vi "AverageLiveSpectra.vi"(6 "Magnitude Averages":u8(slide) scale=1.0..10.0, 9 "old reading":waveform(dbl)[](graph), 10 "new reading":waveform(dbl)[](graph), 11 "Settings":T1 {"Ch_2" min=1 step=1; "Ch_1" min=1 max=100 step=1; "Trigger" items=["Hammer (force)", "Self-tap", "Spacebar"]; "Bandwidth" items=["1 kHz"=1, "5 kHz"=5, "10 kHz"=10, "25 kHz"=25, "50 kHz"=50, "100 kHz"=100]; "High Pass" items=["Off", "13 Hz", "104 Hz"]; "Range" items=["10 mm/s"=1, "20 mm/s"=2, "50 mm/s"=5, "100 mm/s"=10, "200 mm/s"=20, "500 mm/s"=50, "1 m/s"=100, "2 m/s"=200]; "Output" items=["Accelerometer", "Speed (from acceleration)", "Microphone", "Vibrometer", "Piezo"]; "Voltage Cal" format="%#_13g"; "Ch2 Gain" format="%#_13g"; "Ch1 Gain" format="%#_13g"; "Double bounce" min=0.0; "Mic cutoff" min=0.0 format="%#_4g"; "Hammer cutoff" min=0.0 format="%#_4g"; "Freq resolution" min=0.0; "Pre-trigger (s)" format="%#_13g"; "Date" format="%<%H:%M\n%d/%m/%y>T"; "resolution" items=["16 bit"=16, "24 bit"=24, "32 bit"=32]; "Sampling rate" items=["22050 samp/s"=22050, "44100 samp/s"=44100, "48000 samp/s"=48000]}) -> (0 "Hammer":waveform(dbl)(graph), 1 "FIFO out":waveform(dbl)[](array[waveform]), 2 "average spectrum":waveform(dbl), 3 "Power Spectrum":waveform(dbl)(graph), 4 "Microphone":waveform(dbl)(graph), 5 "Cal Hammer":waveform(dbl)[](graph), 7 "cal Mic":waveform(dbl)[](graph))   [LabVIEW 2022 SP3]
uses:
  PreferencesControl.ctl
  <vilib>/Analysis/NI_AALPro.lvlib
panel:
  out "Ch 1":waveform(dbl)(graph)
  # "Hz"
  # "dB"
  # "dB"
  # "sec"
  # "sec"
  # "mV/Pa"
  # "mV/m/s2"
  # "mV/mm/s"
  # "V/N"
  # "sec"
  # "sec"
  # "mV/N"
  # "a.u."
  # "a.u."
  # "sec"
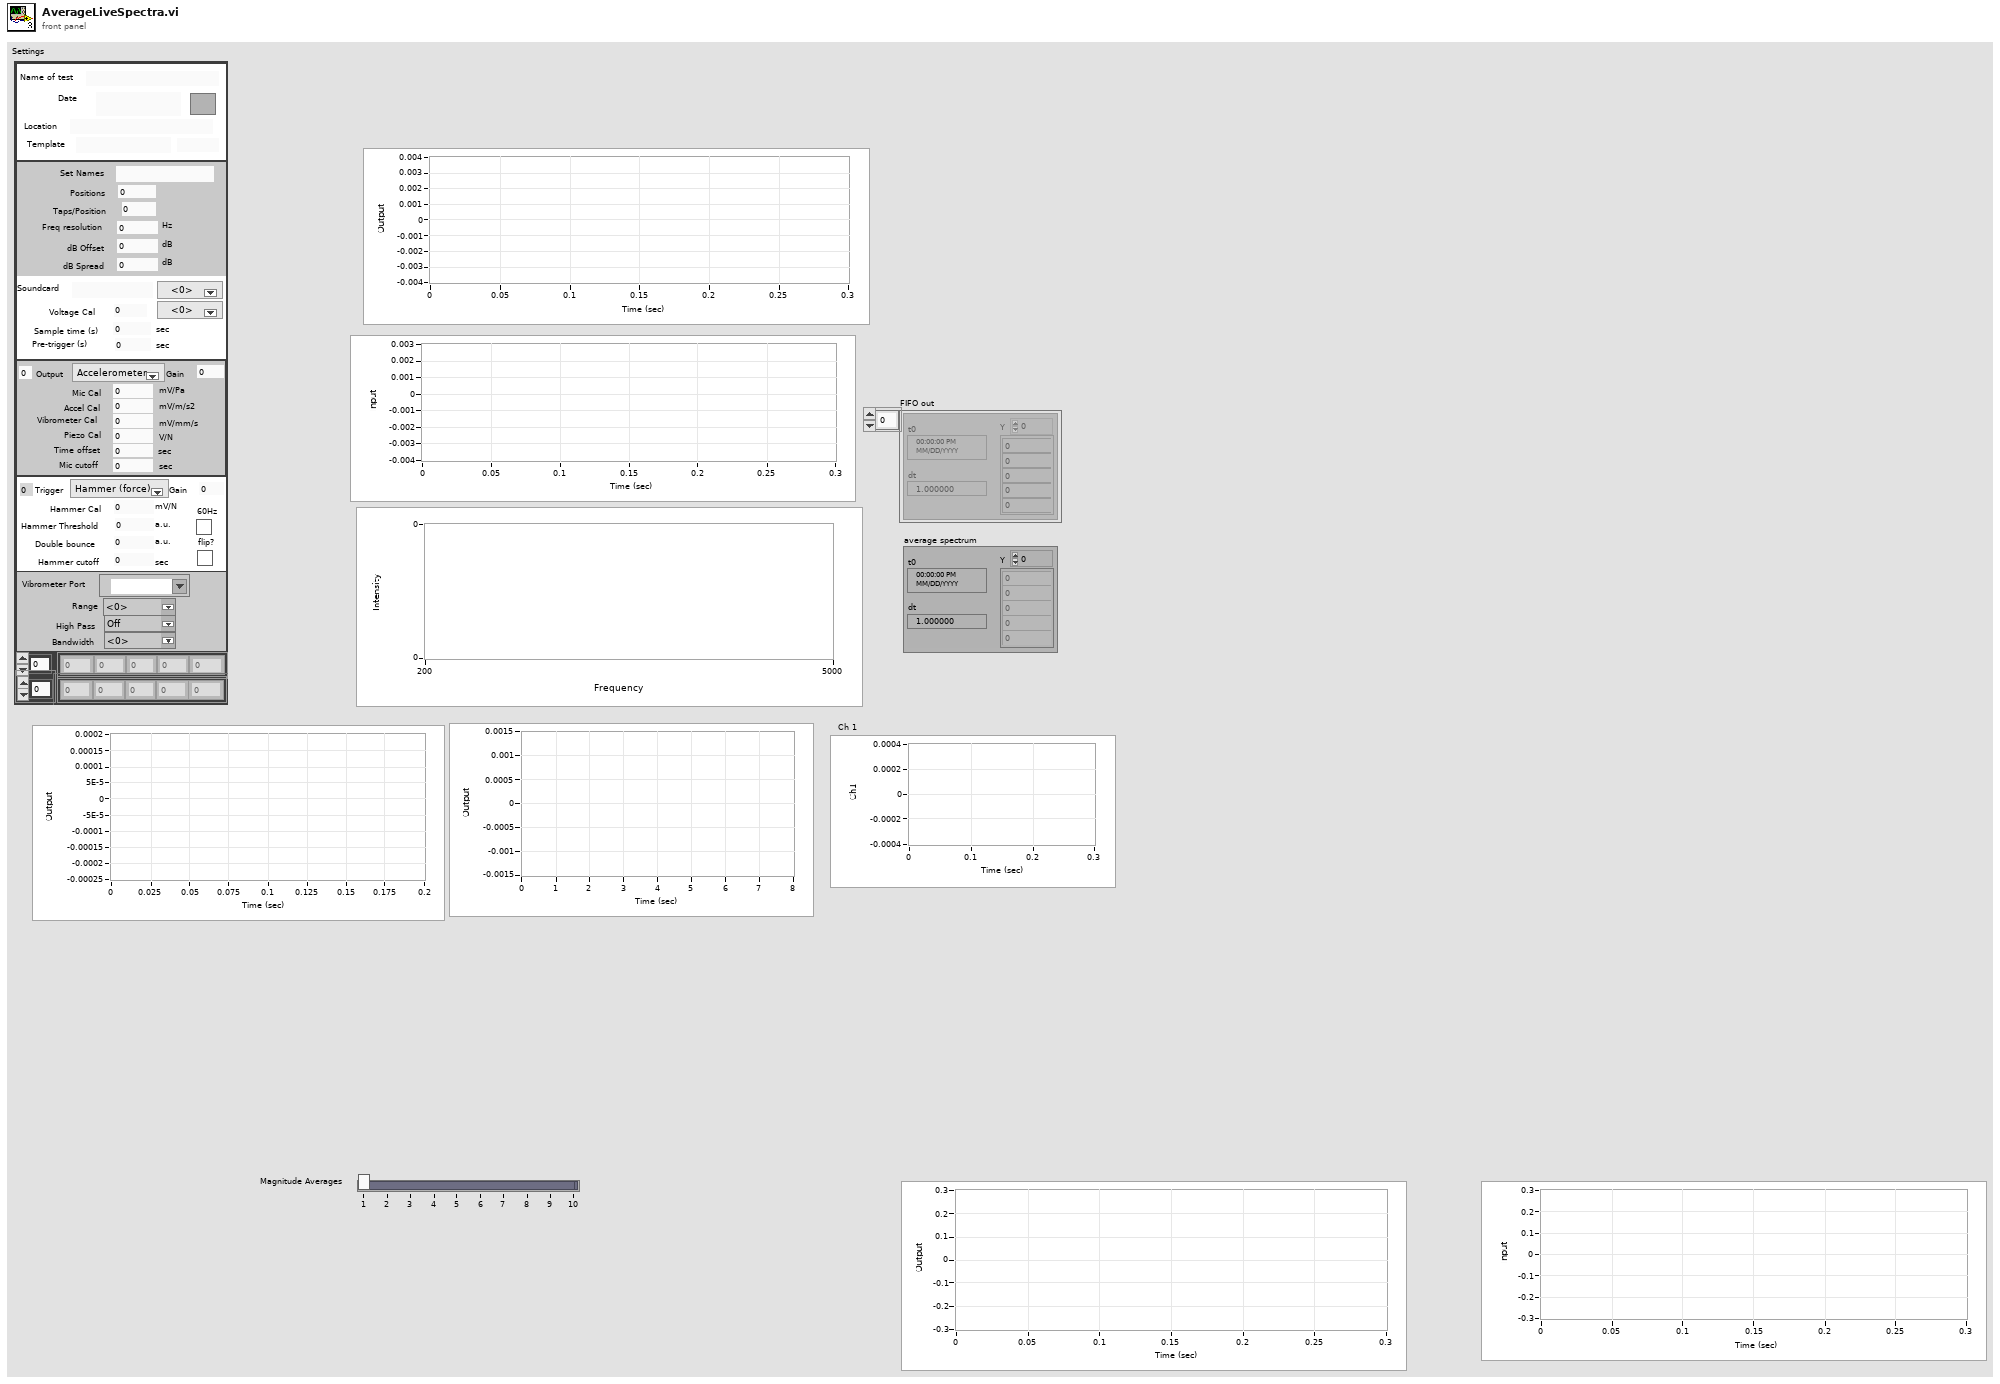
[diagram p1: front panel]
types:
  T1 = typedef "PreferencesControl.ctl" = cluster{"Name of test":string, "Date":timestamp, "Location":string, "Template":string, "Soundcard":string, "resolution":u16, "Sampling rate":u16, "Ch1 Gain ":dbl, "Ch2 Gain":dbl, "Sample time (s)":dbl, "Pre-trigger (s)":dbl, "Hammer Threshold":dbl, "Positions":i16, "Taps/Position":i16, "Set Names":string, "Freq resolution":dbl, "Hammer cutoff":dbl, "Mic cutoff":dbl, "Double bounce ":dbl, "Hammer Cal":dbl, "dB Offset":dbl, "Accel Cal":dbl, "Vibrometer Cal":dbl, "Mic Cal":dbl, "Output":u16, "Voltage Cal":dbl, "Vibrometer Port":refnum<visa-resource-name>, "Range":u16, "High Pass":u16, "Bandwidth":u16, "X Range":cluster{"Minimum":dbl, "Maximum":dbl, "Increment":dbl, "Minor Increment":dbl, "Start":dbl}[], "Y Range":cluster{"Minimum":dbl, "Maximum":dbl, "Increment":dbl, "Minor Increment":dbl, "Start":dbl}[], "dB Spread":dbl, "Trigger":u16, "Ch_1":u8, "Ch_2":u8, "flip?":bool, "60Hz":bool, "Time offset":dbl, "Piezo Cal":dbl, "Default Notes":string}
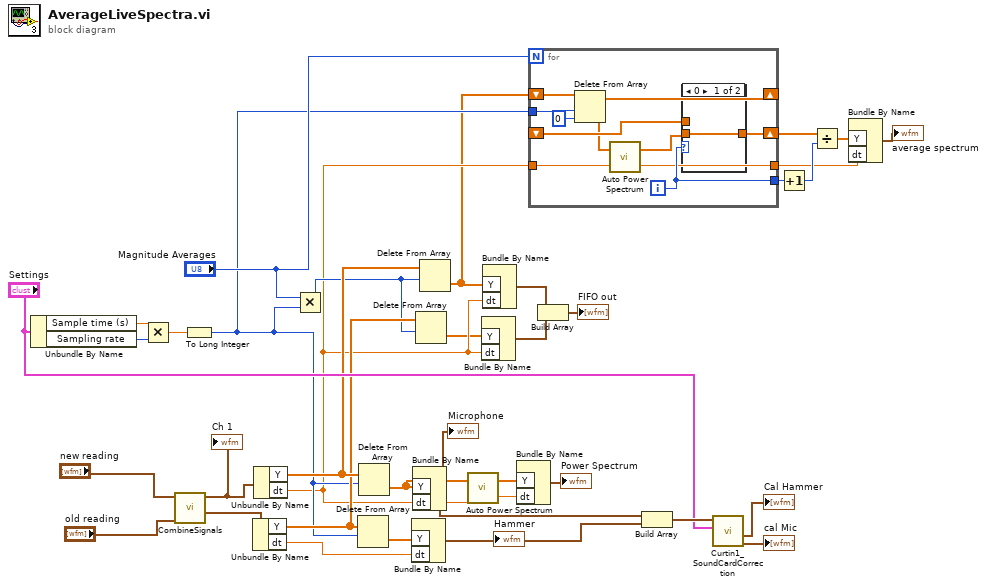
[diagram p0: block diagram]
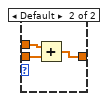
[diagram p2: hidden frame]
diagram:
  n1 = Unbundle By Name("Settings") -> ("Sample time (s)"=w32:dbl, "Sampling rate"=w31:u16)
  n2 = Multiply(x=w32, y=w31) -> (x*y=w30:dbl)
  n3 = call "CombineSignals.vi"("Old signal"="old reading", "New signal"="new reading") -> ("Ch 2"=w1:waveform(dbl), "Ch 1"=w2:waveform(dbl))  [unwired: 8 in]
  "Ch 1" <- w2
  n4 = To Long Integer(number=w30) -> (32bit integer=w12:i32)
  n5 = Unbundle By Name(w1) -> ("Y"=w18:dbl[], "dt"=w25:dbl)
  n6 = Unbundle By Name(w2) -> ("Y"=w19:dbl[], "dt"=w8:dbl)
  n7 = Multiply(x="Magnitude Averages", y=w12) -> (x*y=w17:i32)
  n8 = Delete From Array(array=w18, length=w12) -> (deleted portion=w24:dbl[])  [unwired: 1 in, 1 out]
  n9 = Delete From Array(array=w19, length=w12) -> (deleted portion=w27:dbl[])  [unwired: 1 in, 1 out]
  n10 = Bundle By Name("Y"=w24, "dt"=w25) -> (w22:waveform(dbl))  [unwired: 1 in]
  "Hammer" <- w22
  n11 = Bundle By Name("Y"=w27, "dt"=w8) -> (w23:waveform(dbl))  [unwired: 1 in]
  "Microphone" <- w23
  n12 = Delete From Array(array=w18, length=w17) -> (deleted portion=w6:dbl[])  [unwired: 1 in, 1 out]
  n13 = Delete From Array(array=w19, length=w17) -> (deleted portion=w5:dbl[])  [unwired: 1 in, 1 out]
  n14 = call <vilib>:"Auto Power Spectrum.vi"("dt"=w8, "Signal (V)"=w27) -> ("df"=w28:dbl, "Power Spectrum (V^2 rms)"=w29:dbl[])
  n15 = Bundle By Name("Y"=w6, "dt"=w8) -> (w15:waveform(dbl))  [unwired: 1 in]
  n16 = Bundle By Name("Y"=w5, "dt"=w8) -> (w16:waveform(dbl))  [unwired: 1 in]
  n17 = Bundle By Name("Y"=w29, "dt"=w28) -> (→"Power Spectrum":waveform(dbl))  [unwired: 1 in]
  n18 = for {
    N: "Magnitude Averages" -> [_]
    shift-right: [w47] -> w35
    shift-left: _ -> [w46]
    shift-right: [w42] -> _
    shift-left: w5 -> [w45]
    tunnel: w12 -> [w44]
    tunnel: [w41] -> w11
    tunnel: w8 -> [w38]
    tunnel: [w37] -> w7
    i -> [w41]
    n19 = Delete From Array(array=w45, length=w44, index=0) -> (deleted portion=w40:dbl[], array with subset deleted=w42:dbl[])
    n20 = call <vilib>:"Auto Power Spectrum.vi"("dt"=w38, "Signal (V)"=w40) -> ("df"=w37:dbl, "Power Spectrum (V^2 rms)"=w39:dbl[])
    n21 = case shown="0" w41 {
      tunnel: [w48 w51] -> w47
      tunnel: w39 -> [w48 w49]
      tunnel: w46 -> [_ w50]
      frame 0 {
      }
      frame Default {
        n22 = Add(x=w50, y=w49) -> (x+y=w51:dbl[])
      }
    }
  }
  n23 = Build Array(w16, w15) -> (→"FIFO out":waveform(dbl)[])
  n24 = Build Array(w23, w22) -> (w21:waveform(dbl)[])
  n25 = call "Curtin1_SoundCardCorrection.vi"("Settings"="Settings", "Buffer in"=w21) -> ("Microphone"=→"cal Mic":waveform(dbl)[], "Hammer"=→"Cal Hammer":waveform(dbl)[])  [unwired: 4 in, 4 out]
  n26 = Increment(x=w11) -> (x+1=w10:i32)
  n27 = Divide(x=w35, y=w10) -> (x/y=w9:dbl[])
  n28 = Bundle By Name("Y"=w9, "dt"=w7) -> (→"average spectrum":waveform(dbl))  [unwired: 1 in]
